vi "Published Trace.vi"(8 "error in (no error)":errorcluster, 10 "Trace":refnum<class "Trace.lvclass">, 11 "Trace Listener in":refnum<class "Trace Listener.lvclass">) -> (0 "error out":errorcluster, 3 "Trace Listener out":refnum<class "Trace Listener.lvclass">)   [LabVIEW 2014, in "Robot Actor Framework.lvlib" / "Trace.lvlib" / "Trace Listener.lvclass"]
uses:
  Trace Listener.lvclass
  Trace Class/Trace.lvclass
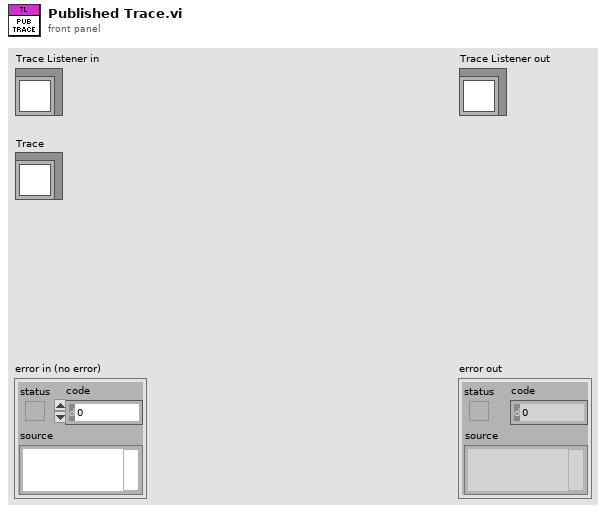
[diagram p1: front panel]
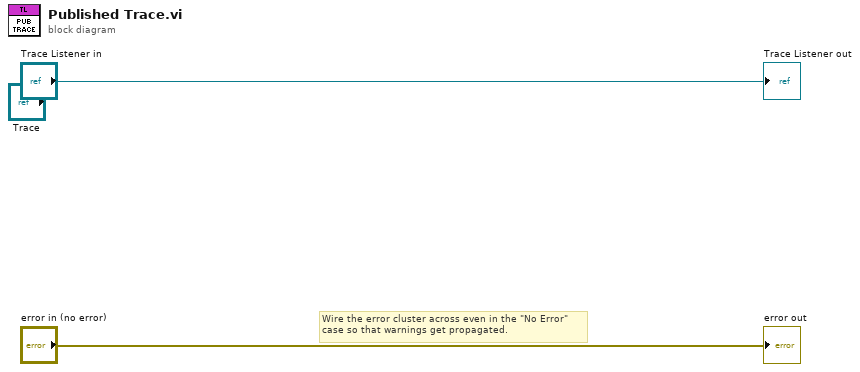
[diagram p0: block diagram]
diagram:
  # "Wire the error cluster across even in the \"No Error\"\ncase so that warnings get propagated."
  "error out" <- "error in (no error)"
  "Trace Listener out" <- "Trace Listener in"
